vi "read37.vi"(0 "VISA资源名称":refnum<visa-resource-name>, 5 "Interval_ms":dbl) -> (2 "SENSOR8":dbl format="%#.2f", 3 "SENSOR6":dbl format="%#.2f", 4 "SENSOR1":dbl format="%#.2g", 6 "SENSOR2":dbl format="%#.2f", 8 "SENSOR3":dbl format="%#.2f", 10 "SENSOR4":dbl format="%#.2f", 13 "SENSOR9":dbl format="%#.2f", 14 "SENSOR7":dbl format="%#.2f", 15 "SENSOR5":dbl format="%#.2f")   [LabVIEW 2017]
uses:
  <vilib>/Instr/_visa.llb/VISA Configure Serial Port (Instr).vi
  <vilib>/addons/Tools/Unicode/UTF8 Tools.lvlib
panel:
  out "sensor1":dbl[](array[numeric])
  out "SENSOR21":dbl[](array[numeric])
  out "SENSOR25":dbl[](array[numeric])
  out "SENDSOR13":dbl[](array[numeric])
  out "SENSOR15":dbl[](array[numeric])
  out "SENSOR5":dbl[](array[numeric])
  out "SNESOR3":dbl[](array[numeric])
  out "SENSOR23":dbl[](array[numeric])
  out "SENSOR11":dbl[](array[numeric])
  out "错误输出 2":errorcluster caption="错误输出"
  in  "?":enum32{"CONTROL", "选项卡 2"}(tab)
  in  "增益选择":u16(ring) items=["±6.144V", "±4.096V", "±2.048V", "±1.024V", "±0.512V", "±0.256V"]
  in  "连接方式":u16(ring) items=["Serial", "WiFi", "Dual"]
  out "数值显示控件 37":dbl
  out "数值显示控件":dbl
  out "数值显示控件 2":dbl
  out "数值显示控件 3":dbl
  out "数值显示控件 5":dbl
  out "数值显示控件 6":dbl
  out "数值显示控件 8":dbl
  out "数值显示控件 9":dbl
  out "数值显示控件 10":dbl
  out "数值显示控件 12":dbl
  out "数值显示控件 13":dbl
  out "数值显示控件 14":dbl
  out "数值显示控件 17":dbl
  out "数值显示控件 18":dbl
  out "数值显示控件 20":dbl
  out "数值显示控件 21":dbl
  out "数值显示控件 22":dbl
  out "数值显示控件 24":dbl
  out "数值显示控件 26":dbl
  out "数值显示控件 27":dbl
  out "数值显示控件 28":dbl
  out "数值显示控件 29":dbl
  out "数值显示控件 30":dbl
  out "数值显示控件 32":dbl
  out "数值显示控件 33":dbl
  out "数值显示控件 34":dbl
  out "数值显示控件 35":dbl
  out "数值显示控件 36":dbl
  out "本次":string
  out "finally":string[][](array[string])
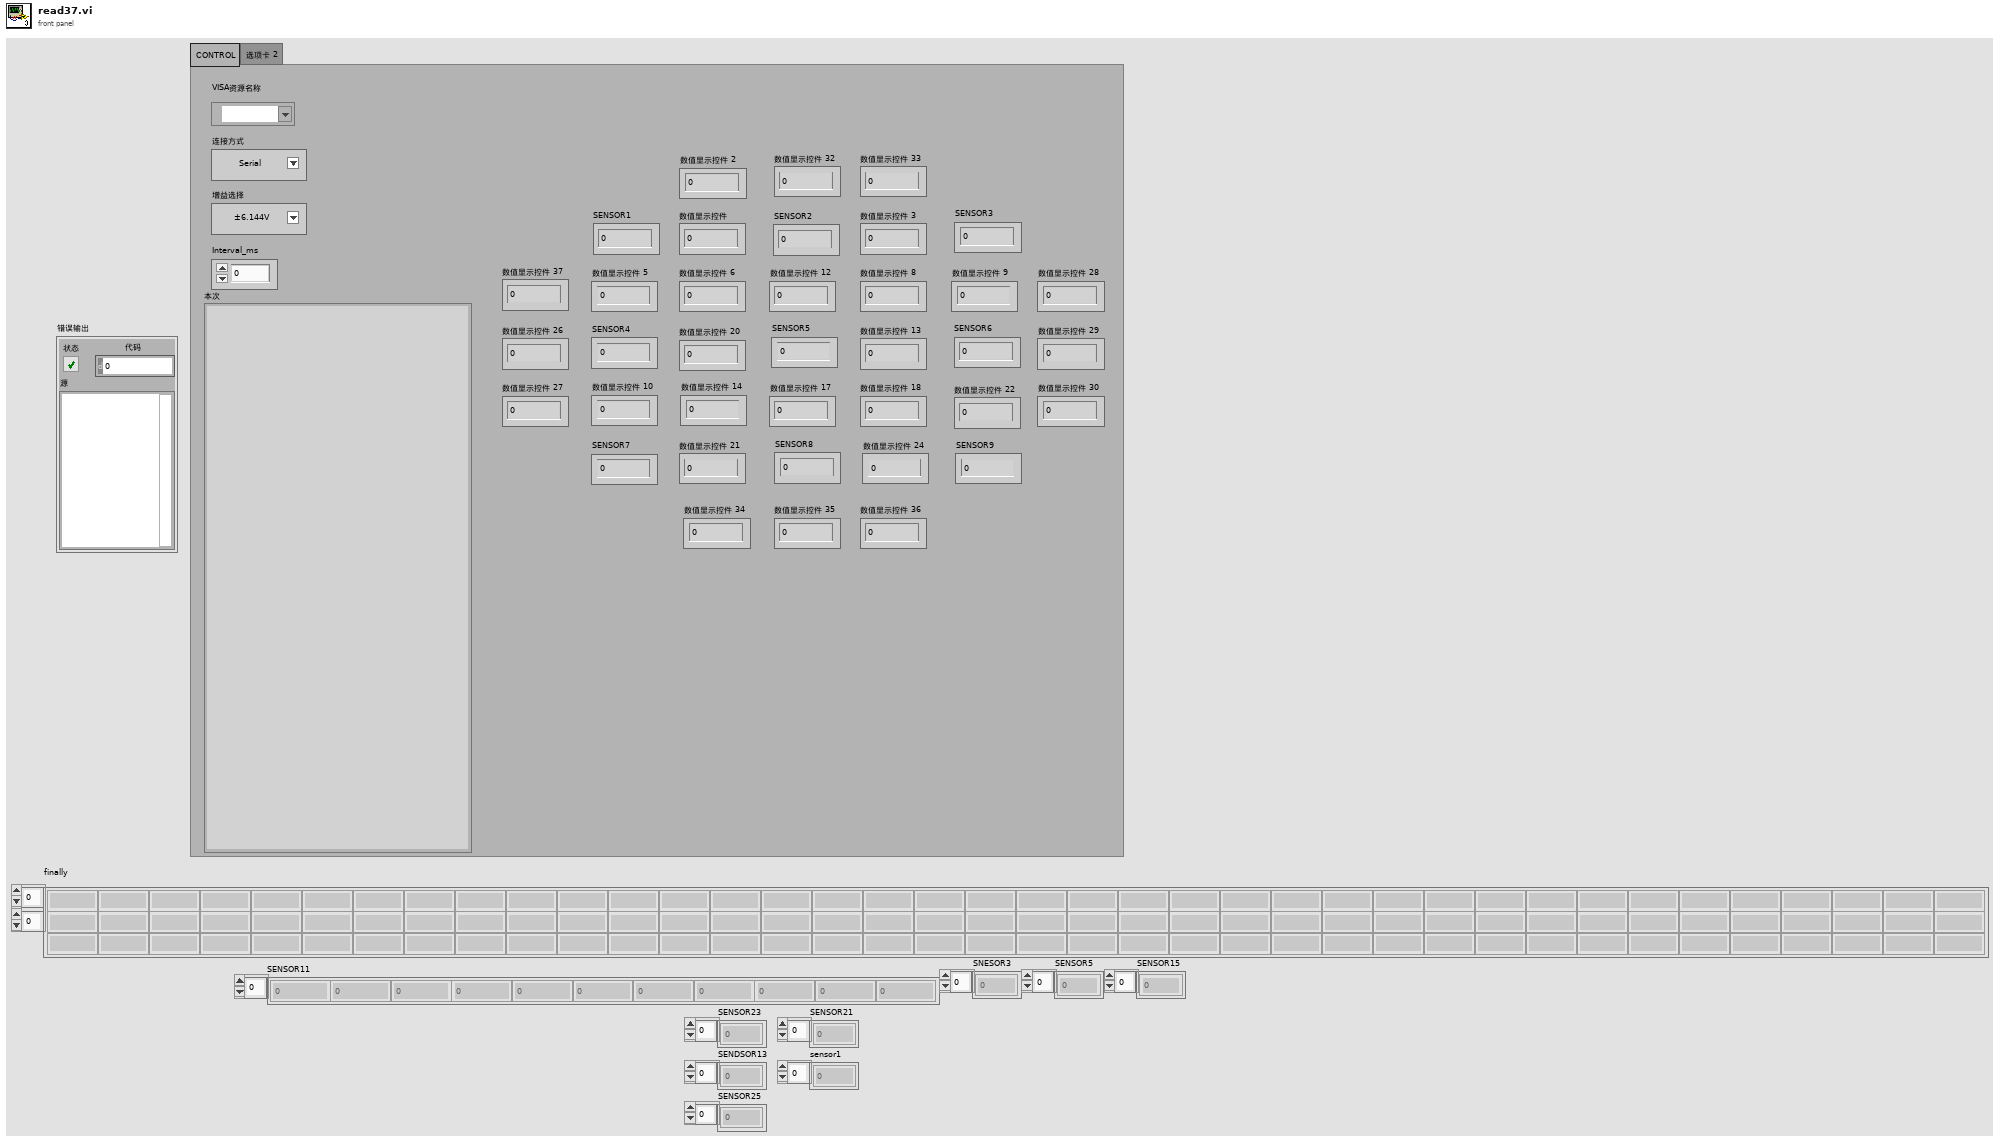
[diagram p1: front panel]
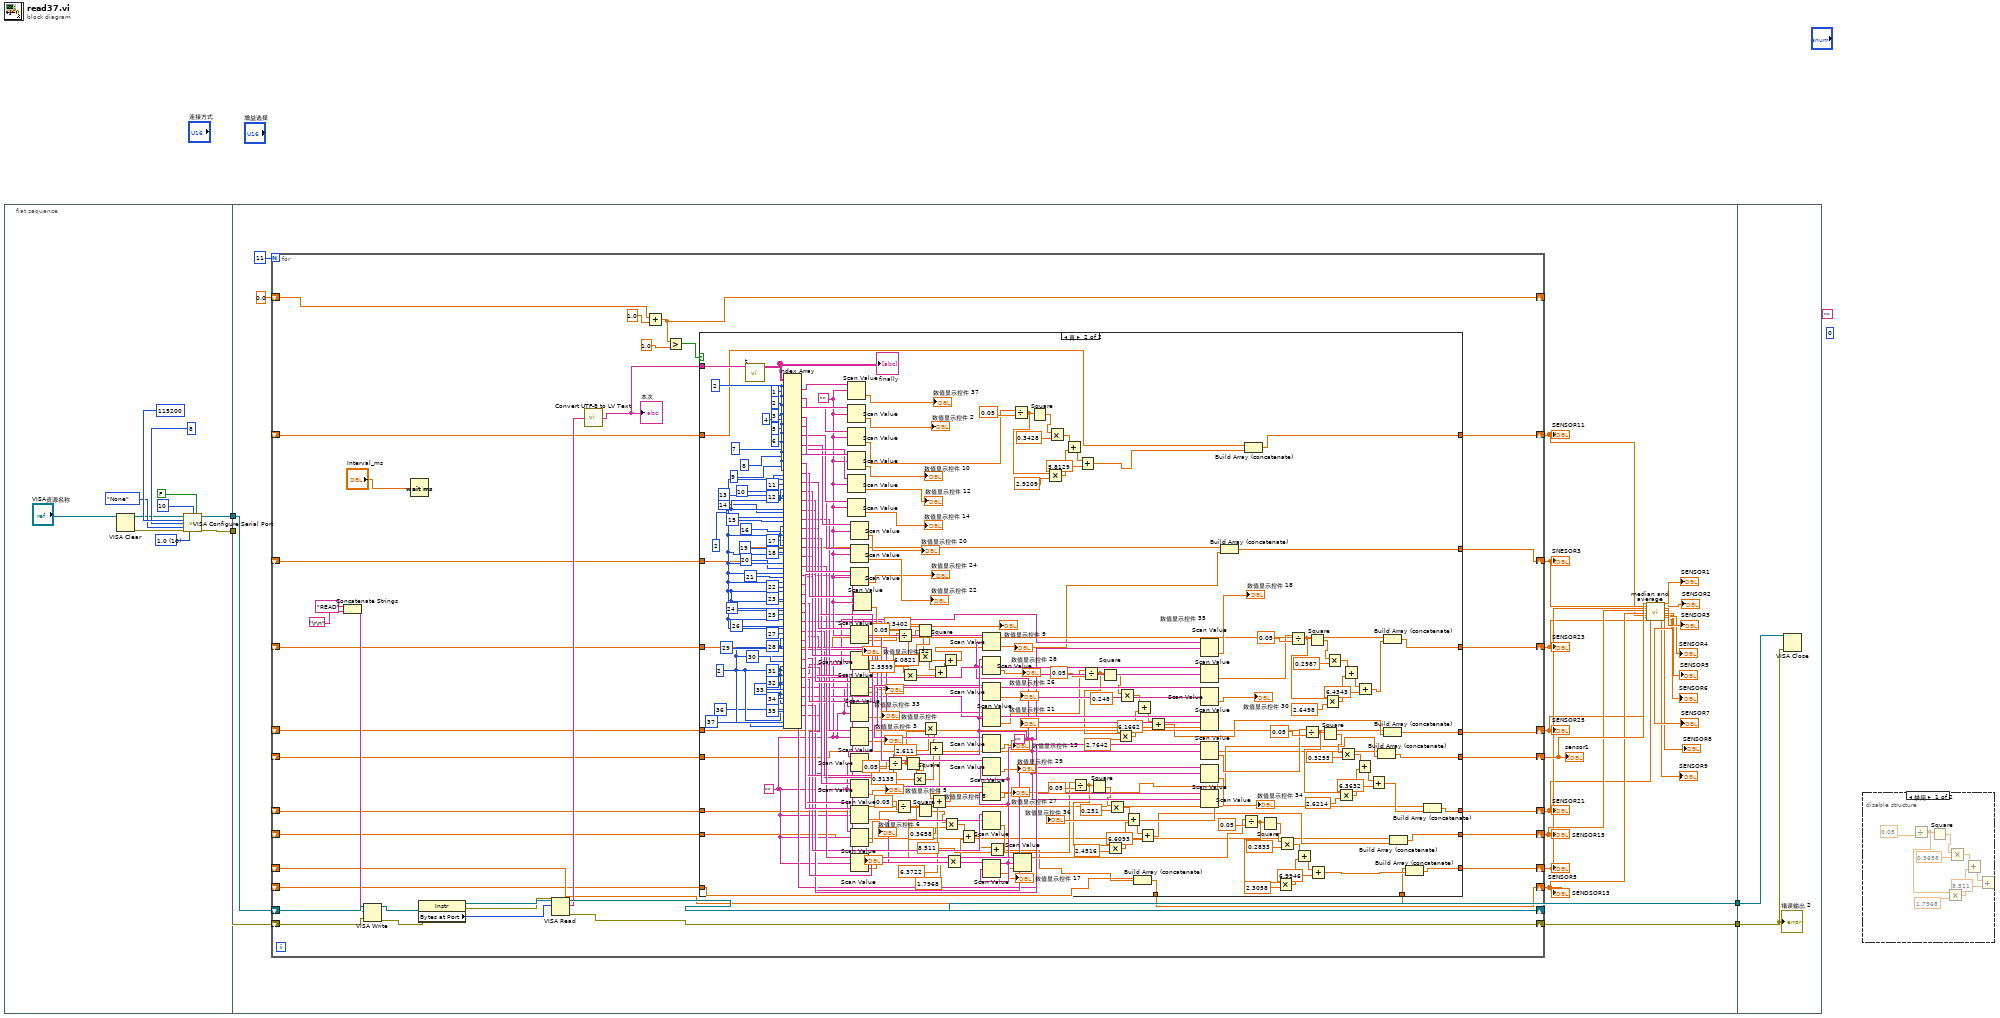
[diagram p0: block diagram]
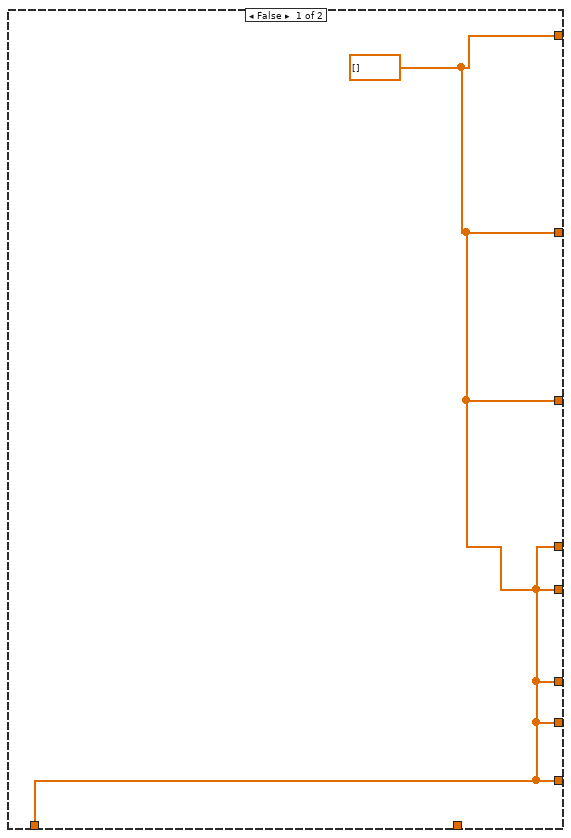
[diagram p3: hidden frame]
diagram:
  (unwired) 0
  (unwired) ""
  n1 = flat-sequence {
    tunnel: [w7] -> w4
    tunnel: [w6] -> w3
    tunnel: w4 -> [w39]
    tunnel: w3 -> [w38]
    tunnel: [w37] -> w2
    tunnel: [w36] -> w1
    tunnel: w2 -> [w307]
    tunnel: w1 -> [w306]
    frame #0 {
      w14 = u16 10 items=["1.0"=10, "1.5"=15, "2.0"=20] ("stop bits (10: 1 bit)")
      n2 = VISA Clear(VISA resource name="VISA资源名称") -> (VISA resource name out=w10:refnum<visa-resource-name>, error out=w9:errorcluster)  [unwired: 1 in]
      n3 = call-poly "VISA Configure Serial Port"("VISA resource name"=w10, "termination char\n(0xA = '\\n' = LF)"=u8 10 ("termination char\n(0xA = '\\n' = LF)"), "Enable Termination\nChar (T)"=FALSE ("Enable Termination\nChar (T)"), "baud rate (9600)"=u32 115200, "data bits (8)"=u16 8, "parity (0:none)"=enum16{"None", "Odd", "Even", "Mark", "Space"}."None", "error in (no error)"=w9, "stop bits (10: 1 bit)"=w14) -> ("VISA resource name out"=w6:refnum<visa-resource-name>, "error out"=w7:errorcluster)  [unwired: 6 in]
    }
    frame #1 {
      n4 = for {
        N: 11 -> [_]
        shift-right: [w74] -> w36
        shift-left: w39 -> [w77]
        shift-right: [w75] -> w37
        shift-left: w38 -> [w76]
        shift-right: [w64] -> _
        shift-left: 0.0 -> [w65]
        shift-right: [w57] -> w28
        shift-left: _ -> [w56]
        shift-right: [w55] -> w26
        shift-left: _ -> [w54]
        shift-right: [w53] -> w32
        shift-left: _ -> [w52]
        shift-right: [w51] -> w31
        shift-left: _ -> [w50]
        shift-right: [w49] -> w30
        shift-left: _ -> [w48]
        shift-right: [w47] -> w29
        shift-left: _ -> [w46]
        shift-right: [w45] -> w27
        shift-left: _ -> [w44]
        shift-right: [w43] -> w25
        shift-left: _ -> [w42]
        shift-right: [w41] -> w33
        shift-left: _ -> [w40]
        n5 = Concatenate Strings("READ" ("字符串"), "\r\n") -> (w73:string)
        n6 = VISA Write(VISA resource name=w76, write buffer=w73, error in (no error)=w77) -> (VISA resource name out=w72:refnum<visa-resource-name>, error out=w71:errorcluster)  [unwired: 1 out]
        n7 = Wait (ms)(milliseconds to wait="Interval_ms") -> ()  [unwired: 1 out]
        n8 = property class="Instr"(reference=w72, error in=w71) -> (reference out=w69:refnum<visa-resource-name>, error out=w68:errorcluster, "Bytes at Port"=w67:u32)
        n9 = VISA Read(VISA resource name=w69, byte count=w67, error in (no error)=w68) -> (VISA resource name out=w75:refnum<visa-resource-name>, read buffer=w66:string, error out=w74:errorcluster)  [unwired: 1 out]
        n10 = call <vilib>:"Convert UTF-8 to LV Text.vi"("UTF-8 Text"=w66) -> ("LV Text"=w58:string)  [unwired: 13 in, 1 out]
        "本次" <- w58
        n11 = Add(x=w65, y=1.0) -> (x+y=w64:dbl)
        n12 = Greater?(x=w64, y=1.0) -> (0:w61:bool)
        n13 = case shown="真" w61 {
          tunnel: w58 -> [_ w106]
          tunnel: [w78 w105] -> w57
          tunnel: w56 -> [_ w104]
          tunnel: [w78 w103] -> w55
          tunnel: w54 -> [_ w101]
          tunnel: [w78 w100] -> w53
          tunnel: w52 -> [_ w98]
          tunnel: [w78 w97] -> w51
          tunnel: w50 -> [_ w95]
          tunnel: [w78 w94] -> w49
          tunnel: w48 -> [_ w92]
          tunnel: [w78 w91] -> w47
          tunnel: w46 -> [_ w89]
          tunnel: [w78 w88] -> w45
          tunnel: w44 -> [_ w86]
          tunnel: [w78 w84] -> w43
          tunnel: w42 -> [_ w83]
          tunnel: [w78 w82] -> w41
          tunnel: w40 -> [_ w80]
          frame False {
            w78 = dbl[] []
          }
          frame True {
            w216 = ""
            w217 = ""
            w248 = 2 ("索引 (行)")
            w274 = 2 ("索引 (行)")
            w244 = ""
            w304 = 2 ("索引 (行)")
            n14 = call "t.vi"("待处理字符串"=w106) -> ("finally"=w305:string[][])  [unwired: 10 in]
            "finally" <- w305
            n15 = Index Array(array=w305, index (row) #1=w304, index (col) #1=1 ("禁用的索引 (列)"), index (row) #2=w304, index (col) #2=2 ("禁用的索引 (列)"), index (row) #3=w304, index (col) #3=3 ("禁用的索引 (列)"), index (row) #4=w304, index (col) #4=4 ("禁用的索引 (列)"), index (row) #5=w304, index (col) #5=5 ("禁用的索引 (列)"), index (row) #6=w304, index (col) #6=6 ("禁用的索引 (列)"), index (row) #7=w304, index (col) #7=7 ("禁用的索引 (列)"), index (row) #8=w304, index (col) #8=8 ("禁用的索引 (列)"), index (row) #9=w304, index (col) #9=9 ("禁用的索引 (列)"), index (row) #10=w304, index (col) #10=10 ("禁用的索引 (列)"), index (row) #11=w274, index (col) #11=11 ("禁用的索引 (列)"), index (row) #12=w274, index (col) #12=12 ("禁用的索引 (列)"), index (row) #13=w274, index (col) #13=13 ("禁用的索引 (列)"), index (row) #14=w274, index (col) #14=14 ("禁用的索引 (列)"), index (row) #15=w274, index (col) #15=15 ("禁用的索引 (列)"), index (row) #16=w274, index (col) #16=16 ("禁用的索引 (列)"), index (row) #17=w274, index (col) #17=17 ("禁用的索引 (列)"), index (row) #18=w274, index (col) #18=18 ("禁用的索引 (列)"), index (row) #19=w274, index (col) #19=19 ("禁用的索引 (列)"), index (row) #20=w274, index (col) #20=20 ("禁用的索引 (列)"), index (row) #21=w274, index (col) #21=21 ("禁用的索引 (列)"), index (row) #22=w274, index (col) #22=22 ("禁用的索引 (列)"), index (row) #23=w274, index (col) #23=23 ("禁用的索引 (列)"), index (row) #24=w274, index (col) #24=24 ("禁用的索引 (列)"), index (row) #25=w274, index (col) #25=25 ("禁用的索引 (列)"), index (row) #26=w274, index (col) #26=26 ("禁用的索引 (列)"), index (row) #27=w274, index (col) #27=27 ("禁用的索引 (列)"), index (row) #28=w248, index (col) #28=28 ("禁用的索引 (列)"), index (row) #29=w248, index (col) #29=29 ("禁用的索引 (列)"), index (row) #30=w248, index (col) #30=30 ("禁用的索引 (列)"), index (row) #31=w248, index (col) #31=31 ("禁用的索引 (列)"), index (row) #32=w248, index (col) #32=32 ("禁用的索引 (列)"), index (row) #33=w248, index (col) #33=33 ("禁用的索引 (列)"), index (row) #34=w248, index (col) #34=34 ("禁用的索引 (列)"), index (row) #35=w248, index (col) #35=35 ("禁用的索引 (列)"), index (row) #36=w248, index (col) #36=36 ("禁用的索引 (列)"), index (row) #37=w248, index (col) #37=37 ("禁用的索引 (列)")) -> (element #1=w296:string, element #2=w295:string, element #3=w294:string, element #4=w293:string, element #5=w292:string, element #6=w291:string, element #7=w290:string, element #8=w289:string, element #9=w285:string, element #10=w284:string, element #11=w245:string, element #12=w243:string, element #13=w242:string, element #14=w241:string, element #15=w240:string, element #16=w239:string, element #17=w238:string, element #18=w237:string, element #19=w236:string, element #20=w235:string, element #21=w234:string, element #22=w233:string, element #23=w232:string, element #24=w231:string, element #25=w230:string, element #26=w229:string, element #27=w228:string, element #28=w227:string, element #29=w226:string, element #30=w225:string, element #31=w224:string, element #32=w223:string, element #33=w222:string, element #34=w221:string, element #35=w220:string, element #36=w219:string, element #37=w218:string)
            n16 = Scan Value(string=w296, format string=w244) -> (value=→"数值显示控件 37":dbl)  [unwired: 1 in, 1 out]
            n17 = Scan Value(string=w295, format string=w244) -> (value=→"数值显示控件 2":dbl)  [unwired: 1 in, 1 out]
            n18 = Scan Value(string=w294, format string=w244) -> (value=w138:dbl)  [unwired: 1 in, 1 out]
            n19 = Scan Value(string=w293, format string=w244) -> (value=→"数值显示控件 10":dbl)  [unwired: 1 in, 1 out]
            n20 = Scan Value(string=w292, format string=w244) -> (value=→"数值显示控件 12":dbl)  [unwired: 1 in, 1 out]
            n21 = Scan Value(string=w291, format string=w244) -> (value=→"数值显示控件 14":dbl)  [unwired: 1 in, 1 out]
            n22 = Scan Value(string=w290, format string=w244) -> (value=→"数值显示控件 20":dbl)  [unwired: 1 in, 1 out]
            n23 = Scan Value(string=w289, format string=w244) -> (value=→"数值显示控件 22":dbl)  [unwired: 1 in, 1 out]
            n24 = Scan Value(string=w285, format string=w244) -> (value=→"数值显示控件 24":dbl)  [unwired: 1 in, 1 out]
            n25 = Scan Value(string=w245, format string=w244) -> (value=w186:dbl)  [unwired: 1 in, 1 out]
            n26 = Scan Value(string=w243, format string=w217) -> (value=→"数值显示控件 32":dbl)  [unwired: 1 in, 1 out]
            n27 = Scan Value(string=w242, format string=w217) -> (value=→"数值显示控件 33":dbl)  [unwired: 1 in, 1 out]
            n28 = Scan Value(string=w241, format string=w217) -> (value=→"数值显示控件":dbl)  [unwired: 1 in, 1 out]
            n29 = Scan Value(string=w240, format string=w217) -> (value=→"数值显示控件 3":dbl)  [unwired: 1 in, 1 out]
            n30 = Scan Value(string=w239, format string=w217) -> (value=w196:dbl)  [unwired: 1 in, 1 out]
            n31 = Scan Value(string=w238, format string=w217) -> (value=→"数值显示控件 5":dbl)  [unwired: 1 in, 1 out]
            n32 = Scan Value(string=w237, format string=w217) -> (value=→"数值显示控件 6":dbl)  [unwired: 1 in, 1 out]
            n33 = Scan Value(string=w236, format string=w217) -> (value=w148:dbl)  [unwired: 1 in, 1 out]
            n34 = Scan Value(string=w235, format string=w217) -> (value=→"数值显示控件 8":dbl)  [unwired: 1 in, 1 out]
            n35 = Scan Value(string=w284, format string=w244) -> (value=→"数值显示控件 35":dbl)  [unwired: 1 in, 1 out]
            n36 = Divide(x=w196, y=0.05) -> (x/y=w191:dbl)
            n37 = Divide(x=w148, y=0.05) -> (x/y=w155:dbl)
            n38 = Divide(x=w186, y=0.05) -> (x/y=w181:dbl)
            n39 = Multiply(x=w181, y=2.5599) -> (x*y=w179:dbl)
            n40 = Square(x=w191) -> (x^2=w194:dbl)
            n41 = Multiply(x=w194, y=0.3135) -> (x*y=w192:dbl)
            n42 = Square(x=w181) -> (x^2=w184:dbl)
            n43 = Multiply(x=w184, y=0.3402) -> (x*y=w182:dbl)
            n44 = Square(x=w155) -> (x^2=w153:dbl)
            n45 = Multiply(x=2.611, y=w191) -> (x*y=w189:dbl)
            n46 = Add(x=w189, y=w192) -> (x+y=w188:dbl)
            n47 = Add(x=w188, y=6.3722) -> (x+y=w81:dbl)
            n48 = Add(x=w182, y=w179) -> (x+y=w178:dbl)
            n49 = Add(x=6.0821, y=w178) -> (x+y=w99:dbl)
            n50 = Multiply(x=w153, y=0.3658) -> (x*y=w154:dbl)
            n51 = Multiply(x=w155, y=1.7968) -> (x*y=w156:dbl)
            n52 = Add(x=w154, y=w156) -> (x+y=w107:dbl)
            n53 = Scan Value(string=w234, format string=w216) -> (value=→"数值显示控件 9":dbl)  [unwired: 1 in, 1 out]
            n54 = Scan Value(string=w233, format string=w216) -> (value=→"数值显示控件 28":dbl)  [unwired: 1 in, 1 out]
            n55 = Scan Value(string=w232, format string=w216) -> (value=→"数值显示控件 26":dbl)  [unwired: 1 in, 1 out]
            n56 = Scan Value(string=w231, format string=w216) -> (value=w128:dbl)  [unwired: 1 in, 1 out]
            n57 = Scan Value(string=w230, format string=w216) -> (value=→"数值显示控件 13":dbl)  [unwired: 1 in, 1 out]
            n58 = Scan Value(string=w229, format string=w216) -> (value=→"数值显示控件 29":dbl)  [unwired: 1 in, 1 out]
            n59 = Scan Value(string=w228, format string=w216) -> (value=→"数值显示控件 27":dbl)  [unwired: 1 in, 1 out]
            n60 = Scan Value(string=w227, format string=w216) -> (value=w157:dbl)  [unwired: 1 in, 1 out]
            n61 = Scan Value(string=w225, format string=w216) -> (value=→"数值显示控件 17":dbl)  [unwired: 1 in, 1 out]
            n62 = Add(x=w107, y=8.511) -> (x+y=w90:dbl)
            n63 = Divide(x=w138, y=0.05) -> (x/y=w143:dbl)
            n64 = Scan Value(string=w226, format string=w216) -> (value=w167:dbl)  [unwired: 1 in, 1 out]
            n65 = Square(x=w143) -> (x^2=w146:dbl)
            n66 = Multiply(x=w143, y=2.9209) -> (x*y=w141:dbl)
            n67 = Multiply(x=w146, y=0.3428) -> (x*y=w144:dbl)
            n68 = Add(x=w144, y=w141) -> (x+y=w140:dbl)
            n69 = Divide(x=w157, y=0.05) -> (x/y=w162:dbl)
            n70 = Add(x=w140, y=5.8129) -> (x+y=w79:dbl)
            n71 = Divide(x=w128, y=0.05) -> (x/y=w134:dbl)
            n72 = Square(x=w162) -> (x^2=w165:dbl)
            n73 = Square(x=w134) -> (x^2=w137:dbl)
            n74 = Multiply(x=w162, y=2.4516) -> (x*y=w160:dbl)
            n75 = Multiply(x=w165, y=0.251) -> (x*y=w163:dbl)
            n76 = Multiply(x=w134, y=2.7642) -> (x*y=w132:dbl)
            n77 = Multiply(x=w137, y=0.248) -> (x*y=w135:dbl)
            n78 = Add(x=w163, y=w160) -> (x+y=w159:dbl)
            n79 = Build Array (concatenate)(w89, w90) -> (w91:dbl[])
            n80 = Add(x=w135, y=w132) -> (x+y=w131:dbl)
            n81 = Add(x=w159, y=6.6093) -> (x+y=w93:dbl)
            n82 = Add(x=w131, y=6.1662) -> (x+y=w87:dbl)
            n83 = Scan Value(string=w224, format string=w216) -> (value=→"数值显示控件 18":dbl)  [unwired: 1 in, 1 out]
            n84 = Scan Value(string=w223, format string=w216) -> (value=w118:dbl)  [unwired: 1 in, 1 out]
            n85 = Scan Value(string=w222, format string=w216) -> (value=→"数值显示控件 30":dbl)  [unwired: 1 in, 1 out]
            n86 = Scan Value(string=w221, format string=w216) -> (value=→"数值显示控件 21":dbl)  [unwired: 1 in, 1 out]
            n87 = Scan Value(string=w220, format string=w216) -> (value=w108:dbl)  [unwired: 1 in, 1 out]
            n88 = Scan Value(string=w219, format string=w216) -> (value=→"数值显示控件 34":dbl)  [unwired: 1 in, 1 out]
            n89 = Scan Value(string=w218, format string=w216) -> (value=→"数值显示控件 36":dbl)  [unwired: 1 in, 1 out]
            n90 = Build Array (concatenate)(w98, w99) -> (w100:dbl[])
            n91 = Divide(x=w167, y=0.05) -> (x/y=w172:dbl)
            n92 = Build Array (concatenate)(w104, w79) -> (w105:dbl[])
            n93 = Square(x=w172) -> (x^2=w175:dbl)
            n94 = Multiply(x=w172, y=2.3058) -> (x*y=w170:dbl)
            n95 = Multiply(x=w175, y=0.2833) -> (x*y=w173:dbl)
            n96 = Divide(x=w118, y=0.05) -> (x/y=w125:dbl)
            n97 = Add(x=w173, y=w170) -> (x+y=w169:dbl)
            n98 = Divide(x=w108, y=0.05) -> (x/y=w115:dbl)
            n99 = Square(x=w125) -> (x^2=w123:dbl)
            n100 = Add(x=w169, y=6.9946) -> (x+y=w96:dbl)
            n101 = Square(x=w115) -> (x^2=w113:dbl)
            n102 = Multiply(x=w125, y=2.6498) -> (x*y=w126:dbl)
            n103 = Multiply(x=w123, y=0.2987) -> (x*y=w124:dbl)
            n104 = Multiply(x=w115, y=2.6214) -> (x*y=w116:dbl)
            n105 = Multiply(x=w113, y=0.3255) -> (x*y=w114:dbl)
            n106 = Add(x=w124, y=w126) -> (x+y=w127:dbl)
            n107 = Add(x=w114, y=w116) -> (x+y=w117:dbl)
            n108 = Add(x=w127, y=6.4343) -> (x+y=w102:dbl)
            n109 = Add(x=w117, y=6.3632) -> (x+y=w85:dbl)
            n110 = Build Array (concatenate)(w80, w81) -> (w82:dbl[])
            n111 = Build Array (concatenate)(w101, w102) -> (w103:dbl[])
            n112 = Build Array (concatenate)(w86, w87) -> (w88:dbl[])
            n113 = Build Array (concatenate)(w92, w93) -> (w94:dbl[])
            n114 = Build Array (concatenate)(w95, w96) -> (w97:dbl[])
            n115 = Build Array (concatenate)(w83, w85) -> (w84:dbl[])
          }
        }
      }
      "SENSOR11" <- w28
      "SENSOR23" <- w26
      "SNESOR3" <- w32
      "SENSOR5" <- w31
      "SENSOR15" <- w30
      "SENDSOR13" <- w29
      "SENSOR25" <- w27
      "SENSOR21" <- w25
      "sensor1" <- w33
      n116 = call "median and average.vi"("sensor 1"=w33, "sensor2"=w32, "sensor3"=w31, "sensor 4"=w30, "sensor 5"=w29, "sensor 6"=w28, "sensor 7"=w27, "sensor 8"=w26, "sensor 9"=w25) -> ("9"=→"SENSOR9":dbl, "1"=→"SENSOR1":dbl, "2"=→"SENSOR2":dbl, "3"=→"SENSOR3":dbl, "4"=→"SENSOR4":dbl, "5"=→"SENSOR5":dbl, "6"=→"SENSOR6":dbl, "7"=→"SENSOR7":dbl, "8"=→"SENSOR8":dbl)  [unwired: 10 in]
    }
    frame #2 {
      n117 = VISA Close(VISA resource name=w307, error in (no error)=w306) -> ()  [unwired: 1 out]
      "错误输出 2" <- w306
    }
  }
  n118 = disable-structure shown="禁用" {
    frame Disabled {
      n119 = Divide(y=0.05) -> (x/y=w312:dbl)  [unwired: 1 in]
      n120 = Square(x=w312) -> (x^2=w315:dbl)
      n121 = Multiply(x=w312, y=1.7968) -> (x*y=w310:dbl)
      n122 = Multiply(x=w315, y=0.3658) -> (x*y=w313:dbl)
      n123 = Add(x=w313, y=w310) -> (x+y=w309:dbl)
      n124 = Add(x=w309, y=8.511) -> ()  [unwired: 1 out]
    }
    frame Enabled {
    }
  }
